vi "GLOBAL DATA INITIALIZE.vi"() -> ()   [LabVIEW 2018]
panel:
  in  "Boolean":bool
  in  "Knob":dbl(knob) scale=0.0..100.0
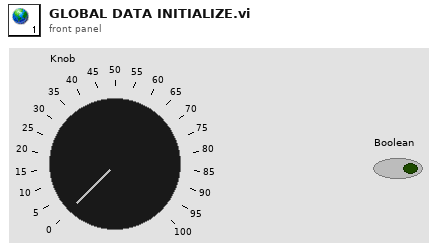
[diagram p1: front panel]
diagram:
